vi "h.ACQ.ParseSensorData.vi"(1 "Raw Sensor Data":u8[](array[numeric])) -> (0 "Sensor Data":T1)   [LabVIEW 2016, in "h.Library.lvlib"]
doc: "This vi parses the data from the h.DAQ.GetPeaks.vi and returns a PeaksData cluster that contains the transfered peaks data.\n\n<b>Data from #GetPeaks</b> - The data returned by the #GetPeaks command\n<b>Peaks Data</b> - cluster containing the peaks data and supporting information"
uses:
  h.Library.lvlib
  CTL/h.ACQ.SensorData.ctl
panel:
  # "Hyperion Parse Sensor Data"
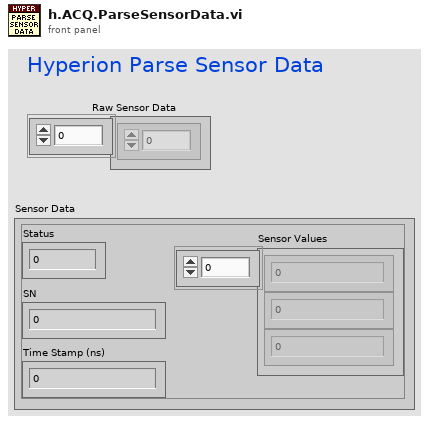
[diagram p1: front panel]
types:
  T1 = typedef "h.Library.lvlib/h.ACQ.SensorData.ctl" = cluster{"SN":u64, "Time Stamp (ns)":u64, "Status":u16, "Sensor Values":dbl[]}
  T2 = enum16{"big-endian, network order", "native, host order", "little-endian"}
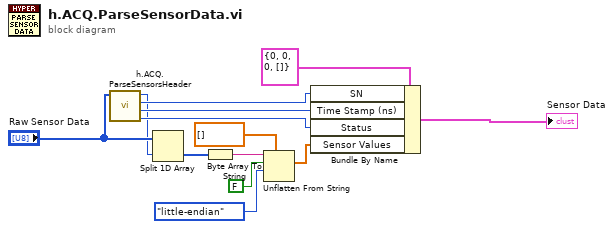
[diagram p0: block diagram]
diagram:
  n1 = call "h.ACQ.ParseSensorsHeader.vi"("Header from #GetPeaks"="Raw Sensor Data") -> ("Status"=w13:u8, "Time Stamp (ns)"=w12:u64, "SN"=w11:u64, "Header Length"=w9:u16)  [unwired: 7 in]
  n2 = Split 1D Array(array="Raw Sensor Data", index=w9) -> (second subarray=w6:u8[])  [unwired: 1 out]
  n3 = Byte Array To String(unsigned byte array=w6) -> (string=w5:string)
  n4 = Unflatten From String(type=dbl[] [], binary string=w5, data includes array or string size? (T)=FALSE, byte order (0:big-endian, network order)=T2."little-endian") -> (value=w1:dbl[])  [unwired: 1 in, 2 out]
  n5 = Bundle By Name(cluster=T1 {"SN"=0, "Time Stamp (ns)"=0, "Status"=0, "Sensor Values"=[]} ("Sensor Data"), "SN"=w11, "Time Stamp (ns)"=w12, "Status"=w13, "Sensor Values"=w1) -> (→"Sensor Data":T1)
